vi "Arm Tester.vi"() -> ()   [LabVIEW 2017]
panel:
  in  "Robot Width":dbl
  in  "Robot Height":dbl
  in  "Pole Height from Ground":dbl
  in  "Forearm Length":dbl
  in  "Backarm Length":dbl
  out "Current Forearm Angle":dbl
  out "Current Backarm Angle":dbl
  out "Current Y":dbl
  out "Current X":dbl
  in  "changeY":dbl(slide) scale=-2.0..2.0
  in  "changeX":dbl(slide) scale=-2.0..2.0
  in  "Forearm Angle":dbl
  in  "Backarm Angle":dbl
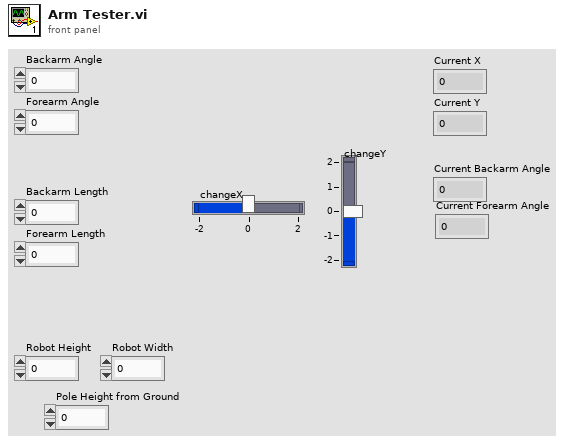
[diagram p1: front panel]
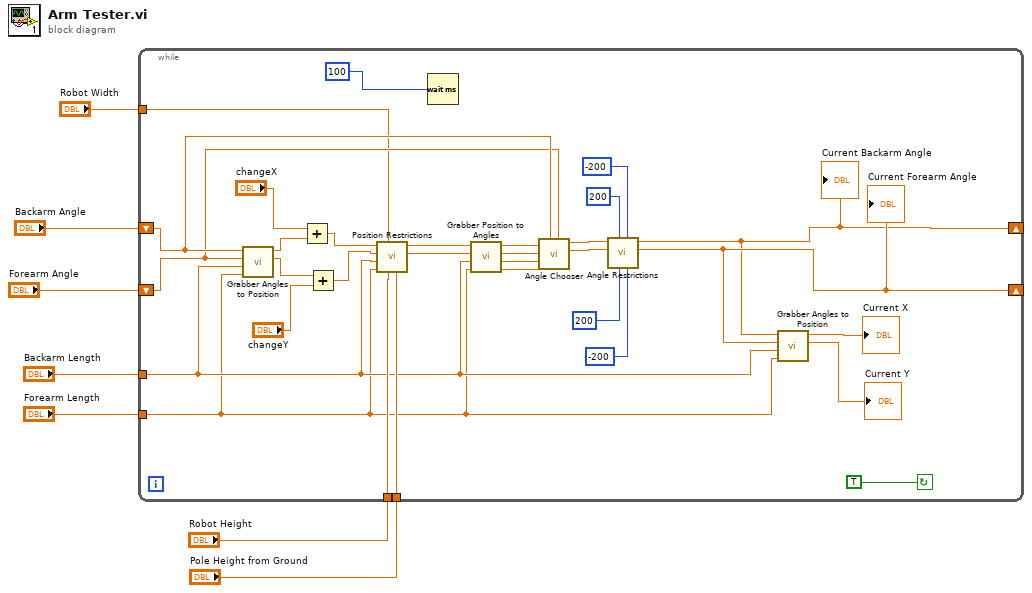
[diagram p0: block diagram]
diagram:
  n1 = while {
    shift-right: [w17] -> _
    shift-left: "Backarm Angle" -> [w26]
    shift-right: [w18] -> _
    shift-left: "Forearm Angle" -> [w25]
    tunnel: "Backarm Length" -> [w10]
    tunnel: "Forearm Length" -> [w9]
    tunnel: "Pole Height from Ground" -> [w14]
    tunnel: "Robot Height" -> [w13]
    tunnel: "Robot Width" -> [w12]
    stop <- TRUE continue-if-true
    n2 = call "Grabber Angles to Position.vi"("Forerm Length"=w9, "Backarm Length"=w10, "Forearm Angle Degrees"=w25, "Backarm Angle Degrees"=w26) -> ("Y Final"=w35:dbl, "X Final"=w36:dbl)  [unwired: 6 in]
    n3 = Add(x="changeX", y=w36) -> (x+y=w34:dbl)
    n4 = Add(x=w35, y="changeY") -> (x+y=w33:dbl)
    n5 = call "Position Restrictions.vi"("Pole Height\nfrom ground"=w14, "Robot Height"=w13, "Robot Width"=w12, "Forearm Length"=w9, "Backarm Length"=w10, "newY"=w33, "newX"=w34) -> ("modified Y"=w31:dbl, "modified X"=w32:dbl)  [unwired: 3 in]
    n6 = Wait (ms)(milliseconds to wait=100) -> ()  [unwired: 1 out]
    n7 = call "Grabber Position to Angles.vi"("Forearm Length"=w9, "Backarm Length"=w10, "Y Initial"=w31, "X Initial"=w32) -> ("Forearm Angle\nDegrees 2"=w27:dbl, "Backarm Angle\nDegrees 2"=w28:dbl, "Forearm Angle\nDegrees 1"=w30:dbl, "Backarm Angle\nDegrees 1"=w29:dbl)  [unwired: 4 in]
    n8 = call "Angle Chooser.vi"("Forearm Angle Initial"=w25, "Backarm Angle Initial"=w26, "Forearm Angle 2"=w27, "Backarm Angle 2"=w28, "Forearm Angle 1"=w30, "Backarm Angle 1"=w29) -> ("final Forearm Angle"=w23:dbl, "final Backarm Angle"=w24:dbl)  [unwired: 4 in]
    n9 = call "Angle Restrictions.vi"("Min Forearm (degrees)"=-200, "Min Backarm (degrees)"=-200, "Max Forearm (degrees)"=200, "Max Backarm (degrees)"=200, "Forearm Angle 1"=w23, "Backarm Angle 1"=w24) -> ("modified Forearm Angle 1"=w18:dbl, "modified Backarm Angle 1"=w17:dbl)  [unwired: 4 in]
    "Current Backarm Angle" <- w17
    "Current Forearm Angle" <- w18
    n10 = call "Grabber Angles to Position.vi"("Forerm Length"=w9, "Backarm Length"=w10, "Forearm Angle Degrees"=w18, "Backarm Angle Degrees"=w17) -> ("Y Final"=→"Current Y":dbl, "X Final"=→"Current X":dbl)  [unwired: 6 in]
  }
